vi "Has Next.vi"(8 "error in (no error)":errorcluster, 11 "Magnetic Field Lakeshore Continuous.lvclass in":refnum<class "Magnetic Field Lakeshore Continuous.lvclass">) -> (0 "error out":errorcluster, 2 "Again?":bool, 3 "Magnetic Field Lakeshore Continuous.lvclass out":refnum<class "Magnetic Field Lakeshore Continuous.lvclass">)   [LabVIEW 2017, in "Magnetic Field Lakeshore Continuous.lvclass"]
doc: "(Dynamic) Return TRUE if this Scanner has not yet completed all steps in its preconfigured Range."
uses:
  Magnetic Field Lakeshore Continuous.lvclass
  Scanner/Scanner.lvclass
  Instruments/Utility Classes/Scannable/Scannable.lvclass
panel:
  out "actual position":dbl
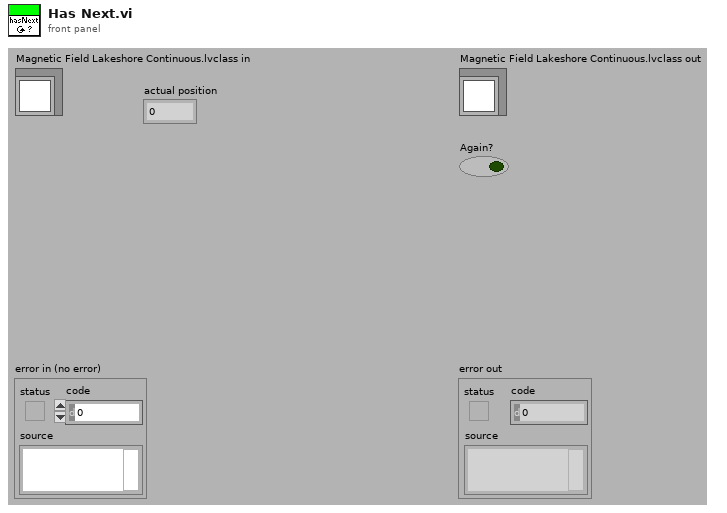
[diagram p1: front panel]
types:
  T1 = typedef "Scanner.lvclass/Range.ctl" = cluster{"xi":dbl, "xf":dbl, "dx":dbl, "Return to...?":bool, "Return to":dbl}
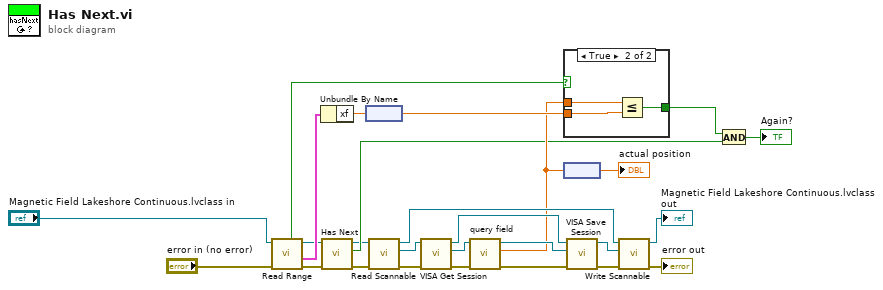
[diagram p0: block diagram]
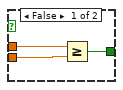
[diagram p2: hidden frame]
diagram:
  n1 = call-dynamic "Read Range.vi"("error in (no error)"="error in (no error)", "Scanner.lvclass in"="Magnetic Field Lakeshore Continuous.lvclass in") -> ("error out"=w2:errorcluster, "Range"=w11:T1, "Scanner.lvclass out"=w5:refnum<class "Magnetic Field Lakeshore Continuous.lvclass">, "Scanning Up?"=w17:bool)  [unwired: 6 out]
  n2 = Unbundle By Name(w11) -> ("xf"=w10:dbl)
  n3 = call-parent "Has Next.vi"("error in (no error)"=w2, "Scanner.lvclass in"=w5) -> ("error out"=w1:errorcluster, "Again?"=w8:bool, "Scanner.lvclass out"=w4:refnum<class "Magnetic Field Lakeshore Continuous.lvclass">)  [unwired: 7 in]
  n4 = node(w10) -> (w18:dbl[unit])
  n5 = call-dynamic "Read Scannable.vi"("error in (no error)"=w1, "Scanner.lvclass in"=w4) -> ("error out"=w27:errorcluster, "Scannable.lvclass"=w22:refnum<class "Scannable.lvclass">, "Scanner.lvclass out"=w23:refnum<class "Magnetic Field Lakeshore Continuous.lvclass">)  [unwired: 7 in]
  n6 = call-dynamic "VISA Get Session.vi"("error in (no error)"=w27, "Instrument.lvclass in"=w22) -> ("error out"=w25:errorcluster, "VISA Resource Name"=w20:refnum<visa-resource-name>, "Instrument.lvclass out"=w16:refnum<class "Scannable.lvclass">)  [unwired: 7 out]
  n7 = call "query field.vi"("error in (no error)"=w25, "VISA session"=w20) -> ("error out"=w26:errorcluster, "Field reading"=w15:dbl[unit], "dup VISA session"=w19:refnum<visa-resource-name>)  [unwired: 7 in]
  n8 = case shown="True" w17 {
    tunnel: w15 -> [w30 w32]
    tunnel: w18 -> [w29 w33]
    tunnel: [w28 w31] -> w9
    frame False {
      n9 = Greater Or Equal?(x=w30, y=w29) -> (x >= y?=w28:bool)
    }
    frame True {
      n10 = Less Or Equal?(x=w32, y=w33) -> (x <= y?=w31:bool)
    }
  }
  n11 = node(w15) -> (→"actual position":dbl)
  n12 = call-dynamic "VISA Save Session.vi"("error in (no error)"=w26, "VISA Resource Name"=w19, "Instrument.lvclass in"=w16) -> ("error out"=w24:errorcluster, "Instrument.lvclass out"=w21:refnum<class "Scannable.lvclass">)  [unwired: 7 out]
  n13 = call-dynamic "Write Scannable.vi"("error in (no error)"=w24, "Scannable.lvclass"=w21, "Scanner.lvclass in"=w23) -> ("error out"=→"error out":errorcluster, "Scanner.lvclass out"=→"Magnetic Field Lakeshore Continuous.lvclass out":refnum<class "Magnetic Field Lakeshore Continuous.lvclass">)  [unwired: 7 in]
  n14 = And(x=w9, y=w8) -> (x .and. y?=→"Again?":bool)
